vi "DecodeFrameHeader.vi"(6 "HeaderLen":i32=2, 8 "ErrorIn":errorcluster, 9 "Header":string="FS", 11 "Frame":string) -> (0 "ErrorOut":errorcluster, 2 "Recognized":bool, 3 "Remainder":string)   [LabVIEW 2016]
doc: "Decode Frame Header. Return information whether it was recognised or not and frame remainder. Error at the input causes no execution. VI throws an error when device has not been recognised."
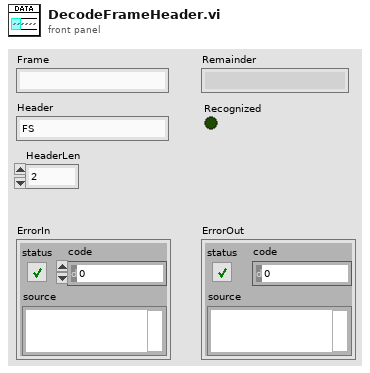
[diagram p1: front panel]
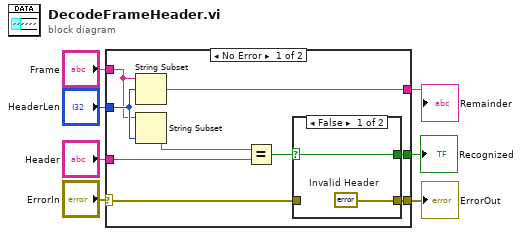
[diagram p0: block diagram]
diagram:
  n1 = case shown="No Error" "ErrorIn" {
    selector: "ErrorIn" -> [w9 w21]
    tunnel: [w16 w21] -> w7
    tunnel: "Header" -> [w14 _]
    tunnel: [w12 _] -> w5
    tunnel: "HeaderLen" -> [w11 _]
    tunnel: "Frame" -> [w10 _]
    tunnel: [w8 _] -> w1
    frame No Error {
      n2 = String Subset(string=w10, offset (0)=w11) -> (substring=w12:string)  [unwired: 1 in]
      n3 = String Subset(string=w10, length (rest)=w11) -> (substring=w13:string)  [unwired: 1 in]
      n4 = Equal?(x=w13, y=w14) -> (x = y?=w15:bool)
      n5 = case shown="False" w15 {
        selector: w15 -> [w17 w19]
        tunnel: w9 -> [_ w20]
        tunnel: [w18 w20] -> w16
        tunnel: [w17 w19] -> w8
        frame False {
          w18 = errorcluster {"status"=TRUE, "code"=2, "source"="Invalid Header"}  # Invalid Header
        }
        frame True {
        }
      }
    }
    frame Error {
    }
  }
  "ErrorOut" <- w7
  "Remainder" <- w5
  "Recognized" <- w1
